vi "light follower new.vi"() -> ()   [LabVIEW 2018]
uses:
  <vilib>/myRIO/Instrument Drivers/Onboard IO/DIO/typedefs/DIO Reference.ctl
  <vilib>/myRIO/Common/Instrument Driver Framework/Utilities/typedefs/myRIO Generic Hardware Reference.ctl
  <vilib>/myRIO/Common/Instrument Driver Framework/Utilities/typedefs/Hardware Version Enum.ctl
  <vilib>/myRIO/Common/Instrument Driver Framework/Utilities/typedefs/myRIO v1.0 Reference.ctl
  <vilib>/myRIO/Common/Instrument Driver Framework/Utilities/typedefs/Generic FPGA Reference.ctl
  <vilib>/myRIO/Common/Instrument Driver Framework/myRIO v1.0/DIO/typedefs/DIO Channels List.ctl
  <vilib>/myRIO/Common/Instrument Driver Framework/myRIO v1.0/DIO/typedefs/DIO Channels Enum.ctl
  <vilib>/userdefined/High Color/nirio_resource_hc.ctl
  <vilib>/myRIO/Instrument Drivers/Onboard IO/PWM/typedefs/PWM Reference.ctl
  <vilib>/myRIO/Common/Instrument Driver Framework/myRIO v1.0/PWM/typedefs/PWM Channels Enum.ctl
  <vilib>/myRIO/Instrument Drivers/Onboard IO/PWM/typedefs/PWM Configuration.ctl
  <vilib>/myRIO/Common/Instrument Driver Framework/Utilities/vis/Is FPGA Ref Available.vi
  <vilib>/myRIO/Common/Instrument Driver Framework/myRIO v1.0/DIO/vis/myRIO v1.1 Open DIO.vi
  <vilib>/myRIO/Instrument Drivers/Onboard IO/DIO/vis/Read.vi
  <vilib>/myRIO/Common/Instrument Driver Framework/myRIO v1.0/PWM/vis/myRIO v1.1 Open PWM.vi
  <vilib>/myRIO/Instrument Drivers/Onboard IO/PWM/vis/Set Duty Cycle and Frequency.vi
  <vilib>/myRIO/Instrument Drivers/Onboard IO/DIO/vis/Write.vi
  <vilib>/myRIO/Common/Instrument Driver Framework/Utilities/vis/Validate Channels.vi
  <vilib>/myRIO/Common/Instrument Driver Framework/myRIO v1.0/DIO/vis/myRIO v1.0 Reserve DIO.vi
  <vilib>/myRIO/Common/Instrument Driver Framework/myRIO v1.0/PWM/vis/myRIO v1.0 Reserve PWM.vi
  <vilib>/myRIO/Common/Instrument Driver Framework/myRIO v1.0/Resource Manager/vis/myRIO v1.0 Reserve Channel List.vi
  <vilib>/myRIO/Common/Instrument Driver Framework/myRIO v1.0/DIO/vis/myRIO v1.0 Build MUX Configuration DIO.vi
  <vilib>/myRIO/Common/Instrument Driver Framework/myRIO v1.0/PWM/vis/myRIO v1.0 Build MUX Configuration PWM.vi
  <vilib>/myRIO/Common/Instrument Driver Framework/myRIO v1.0/Resource Manager/vis/myRIO v1.0 Reserve Channel.vi
  <vilib>/myRIO/Common/Instrument Driver Framework/myRIO v1.0/Resource Manager/vis/myRIO v1.0 Unreserve Channel.vi
  <vilib>/myRIO/Common/Instrument Driver Framework/myRIO v1.0/Resource Manager/vis/myRIO v1.0 Create Configuration List.vi
  <vilib>/myRIO/Common/Instrument Driver Framework/myRIO v1.0/Resource Manager/vis/myRIO v1.0 Build Mutex Name.vi
  <vilib>/Utility/VariantDataType/GetNumericInfo.vi
  <vilib>/Utility/error.llb/Error Cluster From Error Code.vi
  <vilib>/myRIO/Common/Instrument Driver Framework/myRIO v1.0/myRIO v1.1 Open.vi
  <vilib>/myRIO/Common/Instrument Driver Framework/Utilities/vis/IO Manager.vi
  <vilib>/myRIO/Common/Instrument Driver Framework/Utilities/vis/Configuration Manager.vi
  <vilib>/myRIO/Common/Instrument Driver Framework/myRIO v1.0/Resource Manager/vis/myRIO v1.0 Configure IO.vi
  <vilib>/myRIO/Common/Instrument Driver Framework/myRIO v1.0/myRIO v1.0 Close.vi
  <vilib>/myRIO/Common/Instrument Driver Framework/myRIO v1.0/DIO/vis/myRIO v1.0 Read DIO.vi
  <vilib>/myRIO/Common/Instrument Driver Framework/myRIO v1.0/PWM/vis/myRIO v1.0 Write PWM.vi
  <vilib>/myRIO/Common/Instrument Driver Framework/myRIO v1.0/DIO/vis/myRIO v1.0 Write DIO.vi
  <vilib>/myRIO/Express VI/Onboard IO/DI/DI Express VI.xnode
  <vilib>/myRIO/Instrument Drivers/Onboard IO/DIO/vis/myRIO DIO Open.xnode
  <vilib>/myRIO/Express VI/Onboard IO/PWM/PWM Express VI.xnode
  <vilib>/myRIO/Instrument Drivers/Onboard IO/PWM/vis/myRIO PWM Open.xnode
  <vilib>/myRIO/Express VI/Onboard IO/DO/DO Express VI.xnode
  <vilib>/myRIO/Instrument Drivers/Onboard IO/PWM/PWM.lvlib
  <vilib>/myRIO/Instrument Drivers/Onboard IO/DIO/DIO.lvlib
panel:
  out "Boolean 3":bool
  out "Boolean 2":bool
  out "Boolean":bool
  out "error IO":errorcluster
  in  "stop":bool
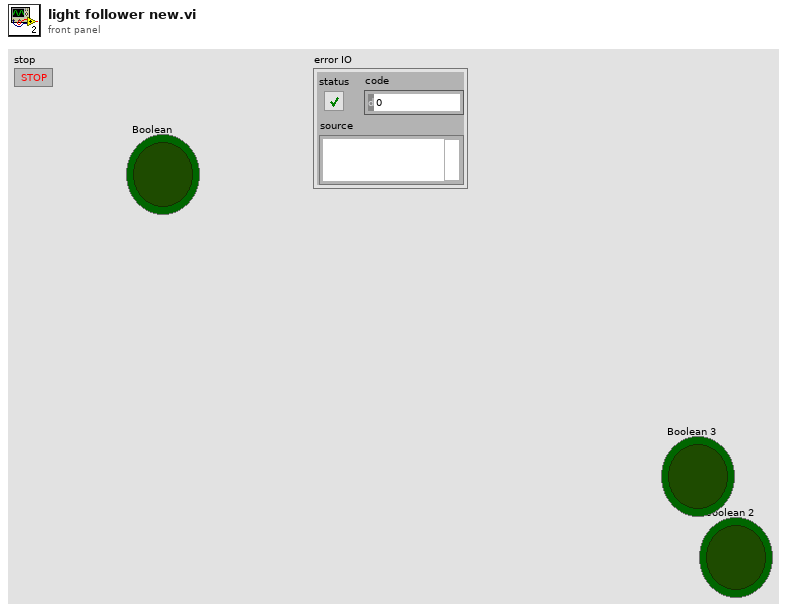
[diagram p1: front panel]
types:
  T1 = typedef "DIO.lvlib/DIO Reference.ctl" = cluster{"myRIO Reference":T2, "DIO Channels List":T6}
  T2 = typedef "myRIO Generic Hardware Reference.ctl" = cluster{"myRIO Model":T3, "myRIO Hardware Reference":T4}
  T3 = typedef "Hardware Version Enum.ctl" = enum16{"Unknown", "myRIO-1900", "myRIO-1950", "roboRIO", "NI ELVIS RIO CM", "ELVIS III"}
  T4 = typedef "myRIO v1.0 Reference.ctl" = cluster{"Generic FPGA Reference":T5, "Allow multiple opens":bool}
  T5 = typedef "Generic FPGA Reference.ctl" = refnum<k20>
  T6 = typedef "DIO Channels List.ctl" = T7[]
  T7 = typedef "DIO Channels Enum.ctl" = enum16{"Not Connected", "C/DIO0", "C/DIO1", "C/DIO2", "C/DIO3", "C/DIO4", "C/DIO5", "C/DIO6", "C/DIO7", "A/DIO0", "A/DIO1", "A/DIO2", "A/DIO3", "A/DIO4", "A/DIO5", "A/DIO6", "A/DIO7", "A/DIO8", "A/DIO9", "A/DIO10", "A/DIO11", "A/DIO12", "A/DIO13", "A/DIO14", "A/DIO15", "A/DIO16", "A/DIO17", "A/DIO18", "A/DIO19", "B/DIO0", "B/DIO1", "B/DIO2", "B/DIO3", "B/DIO4", "B/DIO5", "B/DIO6", "B/DIO7", "B/DIO8", "B/DIO9", "B/DIO10", "B/DIO11", "B/DIO12", "B/DIO13", "B/DIO14", "B/DIO15", "B/DIO16", "B/DIO17", "B/DIO18", "B/DIO19", "LED0", "LED1", "LED2", "LED3", "Button0", "DIO/DIO0", "DIO/DIO1", "DIO/DIO2", "DIO/DIO3", "DIO/DIO4", "DIO/DIO5", "DIO/DIO6", "DIO/DIO7", "DIO/DIO8", "DIO/DIO9", "SPI/CS0", "SPI/CS1", "SPI/CS2", "SPI/CS3", "LED RADIO (Green)", "LED RADIO (Red)", "LED COMM (Green)", "LED COMM (Red)", "LED MODE (Green)", "LED MODE (Red)"}
  T8 = typedef "nirio_resource_hc.ctl" = tag
  T9 = typedef "PWM.lvlib/PWM Reference.ctl" = cluster{"myRIO Reference":T2, "PWM Channels Enum":T10, "PWM Configuration":T11}
  T10 = typedef "PWM Channels Enum.ctl" = enum16{"Not Connected", "C/PWM0", "C/PWM1", "A/PWM0", "A/PWM1", "A/PWM2", "A/PWM3", "A/PWM4", "A/PWM5", "A/PWM6", "A/PWM7", "A/PWM8", "A/PWM9", "A/PWM10", "A/PWM11", "A/PWM12", "A/PWM13", "A/PWM14", "A/PWM15", "A/PWM16", "A/PWM17", "A/PWM18", "A/PWM19", "B/PWM0", "B/PWM1", "B/PWM2", "B/PWM3", "B/PWM4", "B/PWM5", "B/PWM6", "B/PWM7", "B/PWM8", "B/PWM9", "B/PWM10", "B/PWM11", "B/PWM12", "B/PWM13", "B/PWM14", "B/PWM15", "B/PWM16", "B/PWM17", "B/PWM18", "B/PWM19", "PWM/PWM0", "PWM/PWM1", "PWM/PWM2", "PWM/PWM3", "PWM/PWM4", "PWM/PWM5", "PWM/PWM6", "PWM/PWM7", "PWM/PWM8", "PWM/PWM9"}
  T11 = typedef "PWM.lvlib/PWM Configuration.ctl" = cluster{"Frequency":dbl, "Duty Cycle":dbl}
  T12 = enum16{"0", "1", "2", "3", "4", "5", "6", "7", "8", "9", "A", "B", "C", "D", "E", "F", "G", "H", "I", "J", "K", "L", "M", "N", "O", "P", "Q", "R", "S", "T", "U", "V", "W", "X", "Y", "Z", "F1", "F2", "F3", "F4", "F5", "F6", "F7", "F8", "F9", "F10", "F11", "F12", "F13", "F14", "F15", "ADD", "BACK", "BACKSLASH", "CAPITAL", "COMMA", "DECIMAL", "DELETE", "DIVIDE", "DOWN", "END", "EQUALS", "ESCAPE", "GRAVE (`)", "HOME", "INSERT", "LBRACKET", "LCONTROL", "LEFT", "L ALT", "LSHIFT", "LWIN", "MINUS", "MULTIPLY", "NEXT", "NUMLOCK", "NUMPAD_0", "NUMPAD_1", "NUMPAD_2", "NUMPAD_3", "NUMPAD_4", "NUMPAD_5", "NUMPAD_6", "NUMPAD_7", "NUMPAD_8", "NUMPAD_9", "PAUSE", "PERIOD", "PRIOR (PG UP)", "RBRACKET", "RCONTROL", "RETURN", "RIGHT", "R ALT", "RSHIFT", "RWIN", "SCROLL", "SEMICOLON", "SLASH", "SPACE", "SUBTRACT", "TAB", "UP", "ENTER (num pad)", "' (quote)"}[]
  T13 = enum16{"0", "1", "2", "3", "4", "5", "6", "7", "8", "9", "A", "B", "C", "D", "E", "F", "G", "H", "I", "J", "K", "L", "M", "N", "O", "P", "Q", "R", "S", "T", "U", "V", "W", "X", "Y", "Z", "F1", "F2", "F3", "F4", "F5", "F6", "F7", "F8", "F9", "F10", "F11", "F12", "F13", "F14", "F15", "ADD", "BACK", "BACKSLASH", "CAPITAL", "COMMA", "DECIMAL", "DELETE", "DIVIDE", "DOWN", "END", "EQUALS", "ESCAPE", "GRAVE (`)", "HOME", "INSERT", "LBRACKET", "LCONTROL", "LEFT", "L ALT", "LSHIFT", "LWIN", "MINUS", "MULTIPLY", "NEXT", "NUMLOCK", "NUMPAD_0", "NUMPAD_1", "NUMPAD_2", "NUMPAD_3", "NUMPAD_4", "NUMPAD_5", "NUMPAD_6", "NUMPAD_7", "NUMPAD_8", "NUMPAD_9", "PAUSE", "PERIOD", "PRIOR (PG UP)", "RBRACKET", "RCONTROL", "RETURN", "RIGHT", "R ALT", "RSHIFT", "RWIN", "SCROLL", "SEMICOLON", "SLASH", "SPACE", "SUBTRACT", "TAB", "UP", "ENTER (num pad)", "' (quote)"}
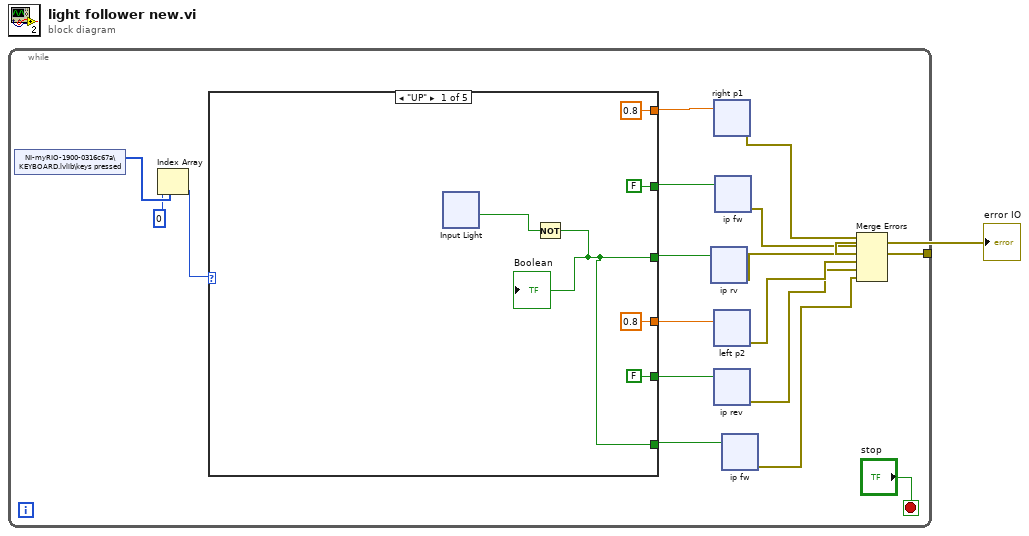
[diagram p0: block diagram]
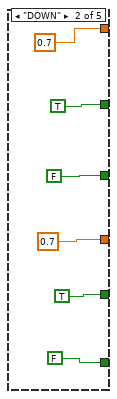
[diagram p2: hidden frame]
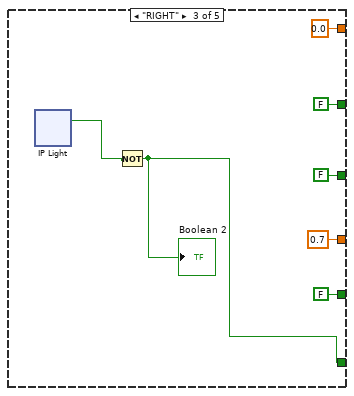
[diagram p3: hidden frame]
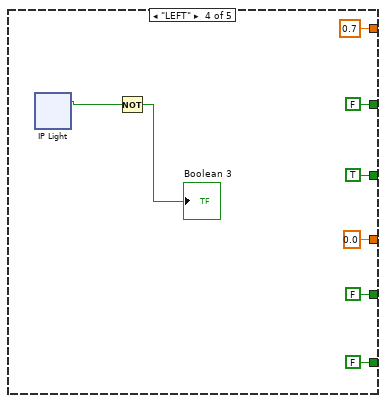
[diagram p4: hidden frame]
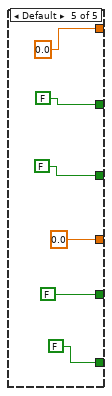
[diagram p5: hidden frame]
diagram:
  n1 = while {
    tunnel: [w18] -> w1
    stop <- "stop" stop-if-true
    n2 = shared-variable "NI-myRIO-1900-0316c67a\\KEYBOARD.lvlib\\keys pressed"() -> (w4:T12)  [unwired: 1 in, 1 out]
    n3 = Index Array "Index Array"(array=w4, index=0) -> (element=w3:T13)
    n4 = case shown="\"UP\"" w3 {
      tunnel: [FALSE ("A/DIO0 (Pin 11)") TRUE ("A/DIO0 (Pin 11)") FALSE ("A/DIO0 (Pin 11)") FALSE ("A/DIO0 (Pin 11)") FALSE ("A/DIO0 (Pin 11)")] -> w10
      tunnel: [w19 FALSE ("A/DIO2 (Pin 15)") FALSE ("A/DIO2 (Pin 15)") TRUE ("A/DIO2 (Pin 15)") FALSE ("A/DIO2 (Pin 15)")] -> w5
      tunnel: [FALSE ("A/DIO4 (Pin 19)") TRUE ("A/DIO4 (Pin 19)") FALSE ("A/DIO4 (Pin 19)") FALSE ("A/DIO4 (Pin 19)") FALSE ("A/DIO4 (Pin 19)")] -> w9
      tunnel: [w19 FALSE ("A/DIO6 (Pin 23)") w67 FALSE ("A/DIO6 (Pin 23)") FALSE ("A/DIO6 (Pin 23)")] -> w8
      tunnel: [0.8 ("Duty Cycle") 0.7 ("Duty Cycle") 0.0 ("Duty Cycle") 0.7 ("Duty Cycle") 0.0 ("Duty Cycle")] -> w7
      tunnel: [0.8 ("Duty Cycle") 0.7 ("Duty Cycle") 0.7 ("Duty Cycle") 0.0 ("Duty Cycle") 0.0 ("Duty Cycle")] -> w6
      frame "UP" {
        n5 = xnode "Input Light"() -> ("B/DIO10 (Pin 31)"=w20:bool)  [unwired: 1 in, 1 out]
        n6 = Not(x=w20) -> (.not. x?=w19:bool)
        "Boolean" <- w19
      }
      frame "DOWN" {
      }
      frame "RIGHT" {
        n7 = xnode "IP Light"() -> ("B/DIO6 (Pin 23)"=w66:bool)  [unwired: 1 in, 1 out]
        n8 = Not(x=w66) -> (.not. x?=w67:bool)
        "Boolean 2" <- w67
      }
      frame "LEFT" {
        n9 = xnode "IP Light"() -> ("B/DIO8 (Pin 27)"=w111:bool)  [unwired: 1 in, 1 out]
        n10 = Not(x=w111) -> (.not. x?=→"Boolean 3":bool)
      }
      frame Default {
      }
    }
    n11 = xnode "ip rv"("A/DIO2 (Pin 15)"=w5) -> ("error out"=w16:errorcluster)  [unwired: 1 in]
    n12 = xnode "right p1"("Duty Cycle"=w7) -> ("error out"=w12:errorcluster)  [unwired: 1 in]
    n13 = xnode "left p2"("Duty Cycle"=w6) -> ("error out"=w15:errorcluster)  [unwired: 1 in]
    n14 = xnode "ip rev"("A/DIO4 (Pin 19)"=w9) -> ("error out"=w14:errorcluster)  [unwired: 1 in]
    n15 = xnode "ip fw"("A/DIO0 (Pin 11)"=w10) -> ("error out"=w11:errorcluster)  [unwired: 1 in]
    n16 = xnode "ip fw"("A/DIO6 (Pin 23)"=w8) -> ("error out"=w13:errorcluster)  [unwired: 1 in]
    n17 = Merge Errors "Merge Errors"(w12, w11, w16, w15, w14, w13) -> (w18:errorcluster)
  }
  "error IO" <- w1
